vi "My Test Path 1.vi"() -> (4 "path":cluster{"X":dbl, "Y":dbl}[](array[cluster])=[{"X"=68.0, "Y"=162.0}, {"X"=69.00000815010367, "Y"=161.99998923782437}, {"X"=70.00000972480896, "Y"=161.999976347877}, {"X"=71.00000589976271, "Y"=161.99997253824438}, {"X"=72.00000258874485, "Y"=161.99997787815312}, {"X"=73.00000345079, "Y"=161.99998501079486}, {"X"=74.0000068882859, "Y"=161.99998763938387}, {"X"=75.00000840196878, "Y"=161.9999856772043}, {"X"=76.00000486810018, "Y"=161.99998146839928}, {"X"=76.99999850673323, "Y"=161.999988282027}, {"X"=77.99998610887653, "Y"=161.9999818517711}, {"X"=78.99999646478759, "Y"=162.00000267244707}, {"X"=79.99997840415463, "Y"=162.00000885555255}, {"X"=80.99999895132635, "Y"=161.99998923381554}, {"X"=82.00001354468957, "Y"=161.99999405963098}, {"X"=83.00000344784759, "Y"=161.99999919986627}, {"X"=83.99999828882413, "Y"=161.99998241356445}, {"X"=85.00000431735211, "Y"=161.9999668723353}, {"X"=86.00000288097867, "Y"=161.99997350483488}, {"X"=86.99998872459678, "Y"=161.99999241855053}, {"X"=87.9999760143925, "Y"=162.00000345578414}, {"X"=88.99997643189944, "Y"=162.0000009425271}, {"X"=89.99998630345718, "Y"=161.99999381646725}, {"X"=90.9999939561318, "Y"=161.99999116346072}, {"X"=91.99999262714807, "Y"=161.9999931418888}, {"X"=92.99998472930808, "Y"=161.99999371224723}, {"X"=93.99997680677556, "Y"=161.9999883239752}, {"X"=94.99997276415951, "Y"=161.9999780285604}, {"X"=95.99997141089959, "Y"=161.99996759354698}, {"X"=96.9999687103102, "Y"=161.99996089233485}, {"X"=97.99996146248489, "Y"=161.99995791073417}, {"X"=98.99994927372327, "Y"=161.9999551589145}, {"X"=99.99993392258945, "Y"=161.99994830747366}, {"X"=100.99991727748362, "Y"=161.99993469594068}, {"X"=101.99989952122124, "Y"=161.99991413134822}, {"X"=102.99987873872229, "Y"=161.99988792137245}, {"X"=103.9998517867924, "Y"=161.99985715375905}, {"X"=104.99981559849208, "Y"=161.99982135962196}, {"X"=105.99976800641726, "Y"=161.9997781373371}, {"X"=106.99970763733822, "Y"=161.99972361903343}, {"X"=107.99963303164812, "Y"=161.99965325382013}, {"X"=108.9995415171625, "Y"=161.99956237048625}, {"X"=109.99942837620452, "Y"=161.99944623098722}, {"X"=110.99928657068887, "Y"=161.99929958047176}, {"X"=111.99910693482916, "Y"=161.9991158860404}, {"X"=112.99887849909402, "Y"=161.99888649051564}, {"X"=113.99858856157087, "Y"=161.9985998295528}, {"X"=114.99822224797997, "Y"=161.99824074152198}, {"X"=115.9977615007, "Y"=161.9977897978924}, {"X"=116.99718360289629, "Y"=161.99722252415475}, {"X"=117.99645940923614, "Y"=161.99650836655314}, {"X"=118.99555141085158, "Y"=161.99560927198883}, {"X"=119.99441164593904, "Y"=161.99447776843783}, {"X"=120.99297933317104, "Y"=161.99305444612483}, {"X"=121.99117799796726, "Y"=161.99126473629778}, {"X"=122.98891180158577, "Y"=161.98901486055888}, {"X"=123.98606076362353, "Y"=161.986186778609}, {"X"=124.98247456617999, "Y"=161.98263189731034}, {"X"=125.97796461438095, "Y"=161.97816322136734}, {"X"=126.97229398048525, "Y"=161.97254552721995}, {"X"=127.96516476508542, "Y"=161.96548302642108}, {"X"=128.95620226610006, "Y"=161.95660384901973}, {"X"=129.94493515646252, "Y"=161.9454405136494}, {"X"=130.93077063623852, "Y"=161.93140534781188}, {"X"=131.9129632409795, "Y"=161.91375956485797}, {"X"=132.8905756447374, "Y"=161.89157437666088}, {"X"=133.86242937483598, "Y"=161.86368210393843}, {"X"=134.8270428306122, "Y"=161.82861471774893}, {"X"=135.7825533379834, "Y"=161.7845265796277}, {"X"=136.72661913769397, "Y"=161.72909731134166}, {"X"=137.656296151911, "Y"=161.65940967633534}, {"X"=138.56788304615887, "Y"=161.57179603949018}, {"X"=139.45672643285548, "Y"=161.4616453205168}, {"X"=140.31697596263942, "Y"=161.3231602811525}, {"X"=141.14127641102294, "Y"=161.14905237654634}, {"X"=141.9203805523161, "Y"=160.93015811791943}, {"X"=142.64266244550262, "Y"=160.65495676309658}, {"X"=143.29350551768428, "Y"=160.30896395626084}, {"X"=143.85453324319775, "Y"=159.87396940554407}, {"X"=144.33953829771096, "Y"=159.3270784741077}, {"X"=144.76407533892638, "Y"=158.69118549740338}, {"X"=145.14051643356743, "Y"=157.98450052521264}, {"X"=145.47870222373302, "Y"=157.22150777649867}, {"X"=145.78645987045533, "Y"=156.4137279844017}, {"X"=146.07001503111763, "Y"=155.5703247516166}, {"X"=146.33431954920553, "Y"=154.69858683020894}, {"X"=146.58331209872674, "Y"=153.804311713029}, {"X"=146.8201254979285, "Y"=152.89211073198948}, {"X"=147.04725160148877, "Y"=151.9656517279783}, {"X"=147.2666724503348, "Y"=151.02785207038988}, {"X"=147.4799645792766, "Y"=150.08103219038838}, {"X"=147.6883819884166, "Y"=149.12703770450125}, {"X"=147.89292210794792, "Y"=148.1673365748784}, {"X"=148.09437832401406, "Y"=147.2030963573212}, {"X"=148.29338166048365, "Y"=146.23524573817878}, {"X"=148.490434054094, "Y"=145.26452333215764}, {"X"=148.68593472749714, "Y"=144.29151668642157}, {"X"=148.8802011973278, "Y"=143.31669313619608}, {"X"=149.0734860209139, "Y"=142.3404244081918}, {"X"=149.2659900797255, "Y"=141.36300622363206}, {"X"=149.45787314223372, "Y"=140.38467382655935}, {"X"=149.64926229227723, "Y"=139.40561433667222}, {"X"=149.84025863118393, "Y"=138.42597661030965}, {"X"=150.0309425916968, "Y"=137.44587907679107}, {"X"=150.22137816587528, "Y"=136.46541595160053}, {"X"=150.41161628040894, "Y"=135.4846621867502}, {"X"=150.60169748399272, "Y"=134.50367742796942}, {"X"=150.79165407815316, "Y"=133.52250916569298}, {"X"=150.98151180977854, "Y"=132.54119523312454}, {"X"=151.1712912238525, "Y"=131.5597657918161}, {"X"=151.36100874751207, "Y"=130.5782449200742}, {"X"=151.55067755589545, "Y"=129.5966518856844}, {"X"=151.74030826197884, "Y"=128.61500216132498}, {"X"=151.92990946964625, "Y"=127.63330823343841}, {"X"=152.11948822355777, "Y"=126.65158025250543}, {"X"=152.30905038047652, "Y"=125.66982656509268}, {"X"=152.4986009191052, "Y"=124.68805415650849}, {"X"=152.68814420223987, "Y"=123.70626902374583}, {"X"=152.87768420503997, "Y"=122.72447649498467}, {"X"=153.0672247233546, "Y"=121.74268151225023}, {"X"=153.25676957468932, "Y"=120.76088889394288}, {"X"=153.4463228022313, "Y"=119.77910359217923}, {"X"=153.63588889114482, "Y"=118.79733095746623}, {"X"=153.82547300704704, "Y"=117.8155770223864}, {"X"=154.01508126883374, "Y"=116.83384881766531}, {"X"=154.2047210708403, "Y"=115.85215473751383}, {"X"=154.39440147210462, "Y"=114.87050497517193}, {"X"=154.58413367347424, "Y"=113.88891205347169}, {"X"=154.77393160725546, "Y"=112.90739147942273}, {"X"=154.96381266982016, "Y"=111.92596255737452}, {"X"=155.15379863545633, "Y"=110.94464940321433}, {"X"=155.34391679987135, "Y"=109.96348221281781}, {"X"=155.53420141424027, "Y"=108.9824988517428}, {"X"=155.72469548596214, "Y"=108.00174685020356}, {"X"=155.9154530412531, "Y"=107.02128590839908}, {"X"=156.10654196859446, "Y"=106.0411910435722}, {"X"=156.29804759239386, "Y"=105.0615565434902}, {"X"=156.49007716464564, "Y"=104.08250093337305}, {"X"=156.68276551085887, "Y"=103.10417321691456}, {"X"=156.87628212740555, "Y"=102.12676071959069}, {"X"=157.0708401038751, "Y"=101.15049894724426}, {"X"=157.26670733996212, "Y"=100.17568397925878}, {"X"=157.46422064703097, "Y"=99.20268804907016}, {"X"=157.66380347623226, "Y"=98.23197913241926}, {"X"=157.86598820594511, "Y"=97.2641455745733}, {"X"=158.07144416142796, "Y"=96.29992705291028}, {"X"=158.28101284145174, "Y"=95.34025350472814}, {"X"=158.49575220617695, "Y"=94.38629406940252}, {"X"=158.7169923575271, "Y"=93.4395186210657}, {"X"=158.94640554290714, "Y"=92.50177513052785}, {"X"=159.18609416689125, "Y"=91.57538692809294}, {"X"=159.43870144319308, "Y"=90.66327498613694}, {"X"=159.7075505107407, "Y"=89.76911165699481}, {"X"=159.9968193357376, "Y"=88.89751395719284}, {"X"=160.31176060504833, "Y"=88.05428657049752}, {"X"=160.65897818419424, "Y"=87.2467273591522}, {"X"=161.04677469031665, "Y"=86.4840114627276}, {"X"=161.4855884733192, "Y"=85.77767420033018}, {"X"=161.98854300405696, "Y"=85.14221819217912}, {"X"=162.5787946654349, "Y"=84.56137735731129}, {"X"=163.23848208022383, "Y"=84.02397719967593}, {"X"=163.95339838834025, "Y"=83.52112957563924}, {"X"=164.7122435173682, "Y"=83.0457648955318}, {"X"=165.50602944140064, "Y"=82.59226003869249}, {"X"=166.32760712611847, "Y"=82.15614239872387}, {"X"=167.1712902626289, "Y"=81.73385448250845}, {"X"=168.03255598675588, "Y"=81.3225666735378}, {"X"=168.907806832346, "Y"=80.92002830499425}, {"X"=169.79418138991397, "Y"=80.52444920440905}, {"X"=170.68940370571264, "Y"=80.13440547450287}, {"X"=171.59166349317843, "Y"=79.7487645548358}, {"X"=172.49952085948908, "Y"=79.36662560632926}, {"X"=173.41183050745178, "Y"=78.98727212124673}, {"X"=174.327681493587, "Y"=78.61013416837174}, {"X"=175.24634921445124, "Y"=78.23475846726825}, {"X"=176.16725737454595, "Y"=77.86078445115463}, {"X"=177.08994754574886, "Y"=77.48792534559058}, {"X"=178.01405510903362, "Y"=77.11595306767585}, {"X"=178.93929006568015, "Y"=76.74468619227494}, {"X"=179.86542173302075, "Y"=76.37398042234163}, {"X"=180.79226662490478, "Y"=76.00372100423053}, {"X"=181.71967881292358, "Y"=75.63381667156611}, {"X"=182.64754222681768, "Y"=75.26419483609259}, {"X"=183.57576453465327, "Y"=74.89479777803842}, {"X"=184.50427229551448, "Y"=74.52557961273004}, {"X"=185.43300710151232, "Y"=74.15650386862356}, {"X"=186.36192249484483, "Y"=73.78754156307251}, {"X"=187.29098151399165, "Y"=73.41866968115622}, {"X"=188.22015475117846, "Y"=73.0498699702523}, {"X"=189.14941881151563, "Y"=72.68112797963819}, {"X"=190.07875508237169, "Y"=72.31243229634924}, {"X"=191.00814874883145, "Y"=71.94377394295269}, {"X"=191.93758801091775, "Y"=71.57514590739979}, {"X"=192.86706346494333, "Y"=71.2065427770372}, {"X"=193.7965676131081, "Y"=70.83796045412751}, {"X"=194.7260944707857, "Y"=70.46939593793292}, {"X"=195.65563925000035, "Y"=70.10084716444203}, {"X"=196.58519810529086, "Y"=69.73231289724501}, {"X"=197.51476793129916, "Y"=69.36379266347686}, {"X"=198.44434620139728, "Y"=68.99528672976086}, {"X"=199.37393083674704, "Y"=68.62679611574056}, {"X"=200.30352009712752, "Y"=68.25832264624329}, {"X"=201.23311248783298, "Y"=67.88986904603817}, {"X"=202.16270667917757, "Y"=67.52143908307681}, {"X"=203.0923014356848, "Y"=67.15303776767598}, {"X"=204.02189555141487, "Y"=66.78467161733339}, {"X"=204.9514877871939, "Y"=66.41634900036124}, {"X"=205.8810768054949, "Y"=66.04808057625571}, {"X"=206.8106610992596, "Y"=65.67987985637998}, {"X"=207.74023891138407, "Y"=65.31176391501316}, {"X"=208.66980814139288, "Y"=64.94375428843537}, {"X"=209.59936623483603, "Y"=64.57587810918638}, {"X"=210.5289100494893, "Y"=64.20816953477639}, {"X"=211.45843569082166, "Y"=63.84067154569948}, {"X"=212.38793830759266, "Y"=63.47343820732114}, {"X"=213.31741183664417, "Y"=63.10653751489689}, {"X"=214.24684868362885, "Y"=62.74005497176472}, {"X"=215.1762393232046, "Y"=62.37409808924055}, {"X"=216.10557179789367, "Y"=62.00880204506117}, {"X"=217.03483108923737, "Y"=61.64433679804054}, {"X"=217.96399832794668, "Y"=61.28091603322033}, {"X"=218.893049801211, "Y"=60.918808408224834}, {"X"=219.82195570474664, "Y"=60.5583516927808}, {"X"=220.75067857391562, "Y"=60.19997054572692}, {"X"=221.67917131148639, "Y"=59.84419886528958}, {"X"=222.60737470843452, "Y"=59.49170788903013}, {"X"=223.53521432742778, "Y"=59.14334152237902}, {"X"=224.46259658498707, "Y"=58.80016075505052}, {"X"=225.38940382604017, "Y"=58.463499502924066}, {"X"=226.31548813152267, "Y"=58.1350348143572}, {"X"=227.2406635330278, "Y"=57.816875135985136}, {"X"=228.1646962247553, "Y"=57.51167128361723}, {"X"=229.08729225766254, "Y"=57.222755958868134}, {"X"=230.00808206824289, "Y"=56.95431915455342}, {"X"=230.92660102773195, "Y"=56.7116286807207}, {"X"=231.84226498804506, "Y"=56.501307417920586}, {"X"=232.7543395373498, "Y"=56.331681889944015}, {"X"=233.6619013470795, "Y"=56.213220501917235}, {"X"=234.56378957593674, "Y"=56.159084508900165}, {"X"=235.47581757318153, "Y"=56.1789733158551}, {"X"=236.3959071900579, "Y"=56.25774374610859}, {"X"=237.3224045737709, "Y"=56.38335165569952}, {"X"=238.25399312262405, "Y"=56.5462180309311}, {"X"=239.18962419123346, "Y"=56.7387248296879}, {"X"=240.1284618987337, "Y"=56.95481403184086}, {"X"=241.0698391351293, "Y"=57.18966879610841}, {"X"=242.0132224503133, "Y"=57.43945994212747}, {"X"=242.9581839777756, "Y"=57.70114441466695}, {"X"=243.9043789152133, "Y"=57.97230512284411}, {"X"=244.8515273772754, "Y"=58.25102372479148}, {"X"=245.79939966309416, "Y"=58.53577966231665}, {"X"=246.74780417191397, "Y"=58.82537013197107}, {"X"=247.69657730385228, "Y"=59.11884677716419}, {"X"=248.64557488216744, "Y"=59.41546578372717}, {"X"=249.59466450805786, "Y"=59.71464870930801}, {"X"=250.54371866635205, "Y"=60.01595208033735}, {"X"=251.49260794795276, "Y"=60.31904399837646}, {"X"=252.44119426804798, "Y"=60.62368671392088}, {"X"=253.38932361110122, "Y"=60.92972410462646}, {"X"=254.33681790036766, "Y"=61.237073437829544}, {"X"=255.28346562912836, "Y"=61.545721033465355}, {"X"=256.22901074261915, "Y"=61.8557215508697}, {"X"=257.17313915653637, "Y"=62.16720085177863}, {"X"=258.1154622177034, "Y"=62.48036262158861}, {"X"=259.0554962517946, "Y"=62.79549909953451}, {"X"=259.99263711307754, "Y"=63.11300646266637}, {"X"=260.92612838644834, "Y"=63.43340567045912}, {"X"=261.85502157156196, "Y"=63.75736987978057}, {"X"=262.7781261608481, "Y"=64.08575987802764}, {"X"=263.6939469841651, "Y"=64.41966939223265}, {"X"=264.60060551769516, "Y"=64.76048265274223}, {"X"=265.49574101314977, "Y"=65.10994724347137}, {"X"=266.37638624564113, "Y"=65.47026607844285}, {"X"=267.2388113433709, "Y"=65.84421334680201}, {"X"=268.0783274798405, "Y"=66.23528052547337}, {"X"=268.88904009480274, "Y"=66.64786014130986}, {"X"=269.663538654216, "Y"=67.08747695473342}, {"X"=270.3925066210792, "Y"=67.56107873490738}, {"X"=271.0642311105297, "Y"=68.07740193204415}, {"X"=271.6639864223094, "Y"=68.64743149218391}, {"X"=272.2048196960084, "Y"=69.29518209109978}, {"X"=272.6987585975971, "Y"=70.00474686539147}, {"X"=273.1553626686934, "Y"=70.7634723293461}, {"X"=273.5822264598023, "Y"=71.56129240099266}, {"X"=273.9853792430144, "Y"=72.39019860829896}, {"X"=274.369602342059, "Y"=73.243818591467}, {"X"=274.73868078126674, "Y"=74.11708071643807}, {"X"=275.0956024977985, "Y"=75.00594714700404}, {"X"=275.4427156017009, "Y"=75.907201326624}, {"X"=275.7818519604259, "Y"=76.81827868519352}, {"X"=276.1144236131408, "Y"=77.73713166155669}, {"X"=276.44149708621063, "Y"=78.66212193584933}, {"X"=276.7638495333805, "Y"=79.59193420810203}, {"X"=277.08200961999404, "Y"=80.52550695592292}, {"X"=277.39628538595093, "Y"=81.46197660468066}, {"X"=277.70678039923763, "Y"=82.40063200083608}, {"X"=278.0133992721301, "Y"=83.34087709099255}, {"X"=278.31584259818425, "Y"=84.28219943838631}, {"X"=278.6135911939319, "Y"=85.22414331912553}, {"X"=278.9058787999922, "Y"=86.16628574108165}, {"X"=279.1916517369793, "Y"=87.10821413934828}, {"X"=279.4695134369017, "Y"=88.04950468195196}, {"X"=279.7376509527375, "Y"=88.98969998242518}, {"X"=279.9937395467305, "Y"=89.92828500925039}, {"X"=280.23482032633075, "Y"=90.86465996768968}, {"X"=280.45714450750785, "Y"=91.79810874355084}, {"X"=280.6559761162, "Y"=92.72776122164835}, {"X"=280.82534273195336, "Y"=93.6525474833089}, {"X"=280.9577211473304, "Y"=94.5711414870313}, {"X"=281.0515205915832, "Y"=95.50585828417438}, {"X"=281.1146393538011, "Y"=96.45334529998074}, {"X"=281.1533609510153, "Y"=97.4109220810787}, {"X"=281.1726848419915, "Y"=98.37643921415695}, {"X"=281.1765895550445, "Y"=99.3481651953131}, {"X"=281.1682420813169, "Y"=100.32469529970321}, {"X"=281.15016455770495, "Y"=101.30487765240419}, {"X"=281.12436701263897, "Y"=102.28775260494962}, {"X"=281.09245315907236, "Y"=103.27250222576978}, {"X"=281.0557048006632, "Y"=104.25840724856269}, {"X"=281.01514929382273, "Y"=105.24480921603354}, {"X"=280.9716136173199, "Y"=106.23107582363777}, {"X"=280.92576789836, "Y"=107.21656764958644}, {"X"=280.8781606813316, "Y"=108.2006044805888}, {"X"=280.82924780249283, "Y"=109.18242955621191}, {"X"=280.77941638057246, "Y"=110.16116965785369}, {"X"=280.72900518551074, "Y"=111.13578925408831}, {"X"=280.67832248114036, "Y"=112.10503590577474}, {"X"=280.62766223286144, "Y"=113.06737439128604}, {"X"=280.5773195876289, "Y"=114.02090592334496}])   [LabVIEW 2018]
uses:
  AutonBuilder/Typedef/Data Point.ctl
panel:
  in  "Data Points":T1[](array[typedef])=[{"X"=68.0, "Y"=162.0, "Theta"=0.0, "Speed %"=0.0, "Disabled?"=FALSE}, {"X"=145.29896907216497, "Y"=162.0, "Theta"=0.0, "Speed %"=0.0, "Disabled?"=FALSE}, {"X"=160.3298969072165, "Y"=84.10452961672475, "Theta"=0.0, "Speed %"=0.0, "Disabled?"=FALSE}, {"X"=234.37113402061857, "Y"=54.75261324041812, "Theta"=0.0, "Speed %"=0.0, "Disabled?"=FALSE}, {"X"=272.78350515463916, "Y"=67.17073170731707, "Theta"=0.0, "Speed %"=0.0, "Disabled?"=FALSE}, {"X"=281.69072164948454, "Y"=94.26480836236934, "Theta"=0.0, "Speed %"=0.0, "Disabled?"=FALSE}, {"X"=280.5773195876289, "Y"=114.02090592334496, "Theta"=0.0, "Speed %"=0.0, "Disabled?"=FALSE}]
  out "Graph":cluster{dbl[], dbl[]}[](graph)=[{[0.0, 33.5, 33.5, 0.0, 0.0], [176.25, 176.25, 147.75, 147.75, 176.25]}, {[68.0, 145.29896907216497, 160.3298969072165, 234.37113402061857, 272.78350515463916, 281.69072164948454, 280.5773195876289], [162.0, 162.0, 84.10452961672475, 54.75261324041812, 67.17073170731707, 94.26480836236934, 114.02090592334496]}, {array[329 elements], array[329 elements]}, {array[329 elements], array[329 elements]}, {array[329 elements], array[329 elements]}]
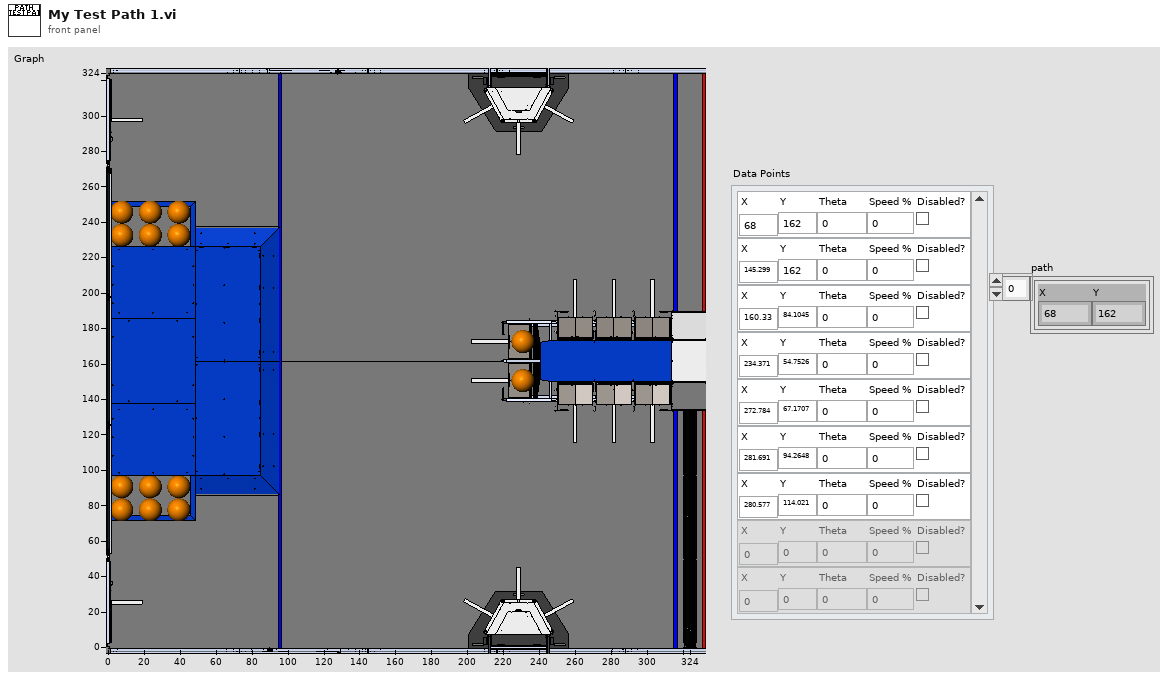
[diagram p1: front panel]
types:
  T1 = typedef "Data Point.ctl" = cluster{"X":dbl, "Y":dbl, "Theta":dbl, "Speed %":dbl, "Disabled?":bool}
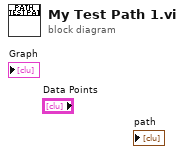
[diagram p0: block diagram]
diagram:
